vi "Test Variant to JSON.vi"() -> ()   [LabVIEW 2011]
uses:
  JSON Value/JSON Value.lvclass
  Variant JSON.lvlib
panel:
  in  "Test Cluster":T1={"T2"="test2", "T1"=456.789, "Nest"={"Enum"=enum."AAA", "NestNest"={"A"="Hi", "B"=2.0, "C"=1}}, "Test Array"=[456.789, 2.0, 3.0], "Boolean"=FALSE}
  out "JSON String":string
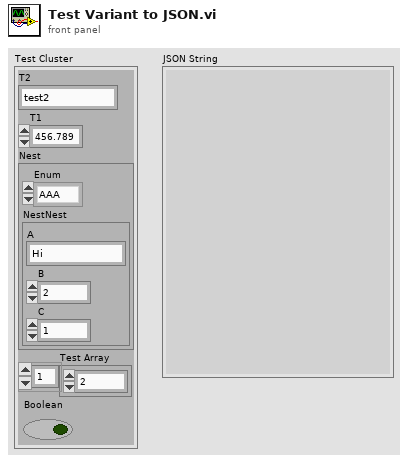
[diagram p1: front panel]
types:
  T1 = cluster{"T2":string, "T1":dbl, "Nest":cluster{"Enum":enum16{"AAA", "BBB", "CCC"}, "NestNest":cluster{"A":string, "B":dbl, "C":i16}}, "Test Array":dbl[], "Boolean":bool}
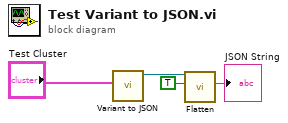
[diagram p0: block diagram]
diagram:
  n1 = call "Variant to JSON.vi"("Variant"="Test Cluster") -> ("JSON Value out"=w2:refnum<class "JSON Value.lvclass">)  [unwired: 9 in, 1 out]
  n2 = call-dynamic "Flatten.vi"("Pretty Print?"=TRUE, "JSON Value in"=w2) -> ("String"=→"JSON String":string)  [unwired: 8 in, 1 out]
